vi "projector_exposure_to_bit_depth.vi"(1 "exp_time_us":i32=8215) -> (0 "BitDepth":i32)   [LabVIEW 2019]
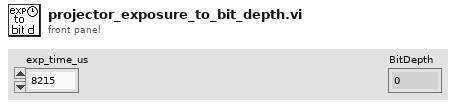
[diagram p1: front panel]
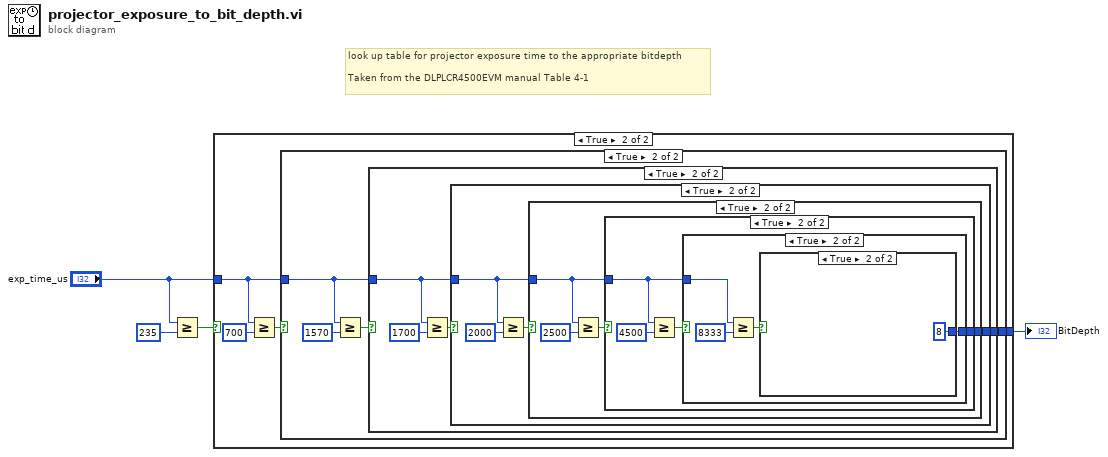
[diagram p0: block diagram]
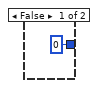
[diagram p2: hidden frame]
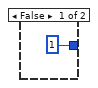
[diagram p3: hidden frame]
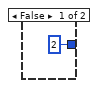
[diagram p4: hidden frame]
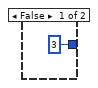
[diagram p5: hidden frame]
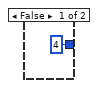
[diagram p6: hidden frame]
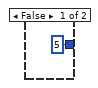
[diagram p7: hidden frame]
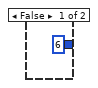
[diagram p8: hidden frame]
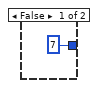
[diagram p9: hidden frame]
diagram:
  # "look up table for projector exposure time to the appropriate bitdepth\n\nTaken from the DLPLCR4500EVM manual Table 4-1"
  n1 = Greater Or Equal?(x="exp_time_us", y=235) -> (x >= y?=w3:bool)
  n2 = case shown="True" w3 {
    tunnel: "exp_time_us" -> [_ w6]
    tunnel: [0 ("BitDepth") w7] -> w1
    frame False {
    }
    frame True {
      n3 = Greater Or Equal?(x=w6, y=700) -> (x >= y?=w8:bool)
      n4 = case shown="True" w8 {
        tunnel: [1 ("BitDepth") w12] -> w7
        tunnel: w6 -> [_ w11]
        frame False {
        }
        frame True {
          n5 = Greater Or Equal?(x=w11, y=1570) -> (x >= y?=w13:bool)
          n6 = case shown="True" w13 {
            tunnel: [2 ("BitDepth") w17] -> w12
            tunnel: w11 -> [_ w16]
            frame False {
            }
            frame True {
              n7 = Greater Or Equal?(x=w16, y=1700) -> (x >= y?=w18:bool)
              n8 = case shown="True" w18 {
                tunnel: [3 ("BitDepth") w22] -> w17
                tunnel: w16 -> [_ w21]
                frame False {
                }
                frame True {
                  n9 = Greater Or Equal?(x=w21, y=2000) -> (x >= y?=w23:bool)
                  n10 = case shown="True" w23 {
                    tunnel: [4 ("BitDepth") w26] -> w22
                    tunnel: w21 -> [_ w27]
                    frame False {
                    }
                    frame True {
                      n11 = Greater Or Equal?(x=w27, y=2500) -> (x >= y?=w28:bool)
                      n12 = case shown="True" w28 {
                        tunnel: w27 -> [_ w32]
                        tunnel: [5 ("BitDepth") w31] -> w26
                        frame False {
                        }
                        frame True {
                          n13 = Greater Or Equal?(x=w32, y=4500) -> (x >= y?=w33:bool)
                          n14 = case shown="True" w33 {
                            tunnel: w32 -> [_ w38]
                            tunnel: [6 ("BitDepth") w36] -> w31
                            frame False {
                            }
                            frame True {
                              n15 = Greater Or Equal?(x=w38, y=8333) -> (x >= y?=w37:bool)
                              n16 = case shown="True" w37 {
                                tunnel: [7 ("BitDepth") 8 ("BitDepth")] -> w36
                                frame False {
                                }
                                frame True {
                                }
                              }
                            }
                          }
                        }
                      }
                    }
                  }
                }
              }
            }
          }
        }
      }
    }
  }
  "BitDepth" <- w1
